vi "Position Popup.vi"(0 "Cluster Referenz":refnum<vi>, 11 "error in (no error)":errorcluster caption="Fehler (Eingang, kein Fehler)", 13 "Aktion":enum16{"Init", "lesen", "schreiben"}(ring)) -> (4 "Position":T1 caption="x-y", 15 "error out":errorcluster caption="Fehler (Ausgang)")   [LabVIEW 2020, in "CalGas Aufschaltung.lvlib"]
uses:
  CalGas Aufschaltung.lvlib
  Funktionstasten/Funktionstasten.ctl
  <vilib>/Utility/miscctls.llb/LVPositionTypeDef.ctl
  Funktionstasten/Funktionstasten.lvlib
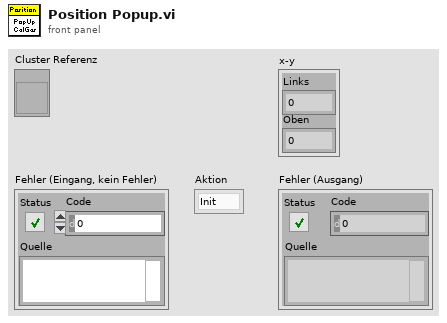
[diagram p1: front panel]
types:
  T1 = typedef "LVPositionTypeDef.ctl" = cluster{"Left":i32, "Top":i32}
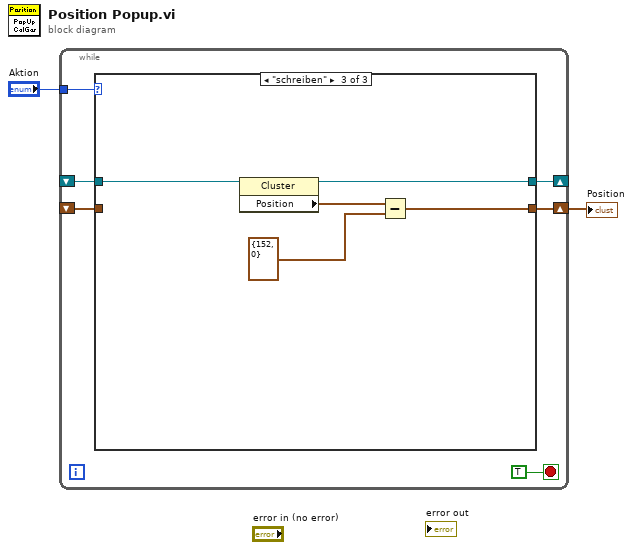
[diagram p0: block diagram]
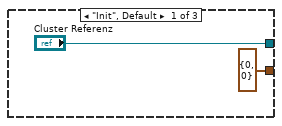
[diagram p2: hidden frame]
diagram:
  n1 = while {
    tunnel: "Aktion" -> [w7]
    shift-right: [w6] -> _
    shift-left: _ -> [w5]
    shift-right: [w4] -> w1
    shift-left: _ -> [w3]
    stop <- TRUE stop-if-true
    n2 = case shown="\"schreiben\"" w7 {
      tunnel: ["Cluster Referenz" w12 w16] -> w6
      tunnel: w5 -> [_ w12 w17]
      tunnel: [T1 {"Left"=0, "Top"=0} ("Position") w11 w13] -> w4
      tunnel: w3 -> [_ w11 _]
      frame "Init", Default {
      }
      frame "lesen" {
      }
      frame "schreiben" {
        n3 = property class="Cluster"(reference=w17) -> (reference out=w16:refnum<vi>, "Position"=w15:T1)  [unwired: 1 in, 1 out]
        n4 = Subtract(x=w15, y=T1 {"Left"=152, "Top"=0} ("Position")) -> (x-y=w13:T1)
      }
    }
  }
  "Position" <- w1
